vi "Extract Msg Segments.vi"(7 "Start Index":i32, 8 "error in (no error)":errorcluster, 10 "Segments in":T1[](array[typedef]), 11 "ProtoParser in":refnum<class "ProtoParser.lvclass">) -> (0 "error out":errorcluster, 1 "Message Segments":T1[](array[typedef]), 2 "Remaining":T1[](array[typedef]), 3 "ProtoParser out":refnum<class "ProtoParser.lvclass">, 5 "Next Index":i32)   [LabVIEW 2024, in "LV-Protoc.lvlib" / "ProtoParser.lvclass"]
uses:
  ProtoParser.lvclass
  ProtoParser.lvclass/ProtoParser.ctl
  Segment Type.ctl
  LV-Protoc.lvlib
  Raw Segment.ctl
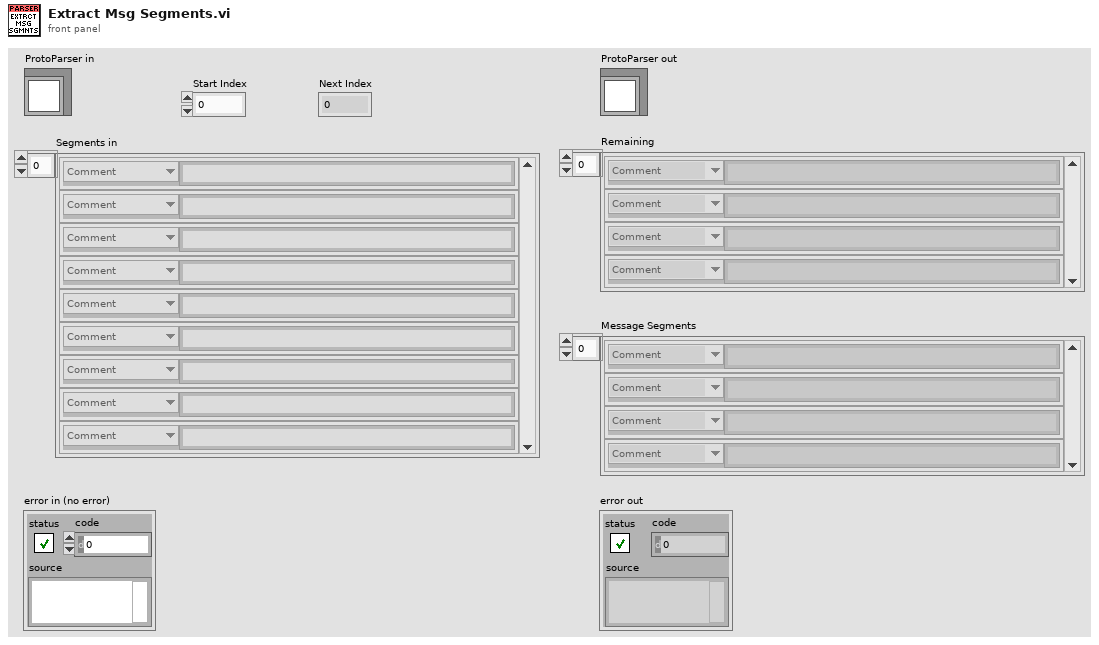
[diagram p1: front panel]
types:
  T1 = typedef "LV-Protoc.lvlib/Raw Segment.ctl" = cluster{"Type":T2, "Text":string}
  T2 = typedef "LV-Protoc.lvlib/Segment Type.ctl" = enum16{"Comment", "Message Open", "Enum Open", "Message Close", "Enum Close", "Field", "Syntax", "Import", "Enum Value", "Package", "Reserved"}
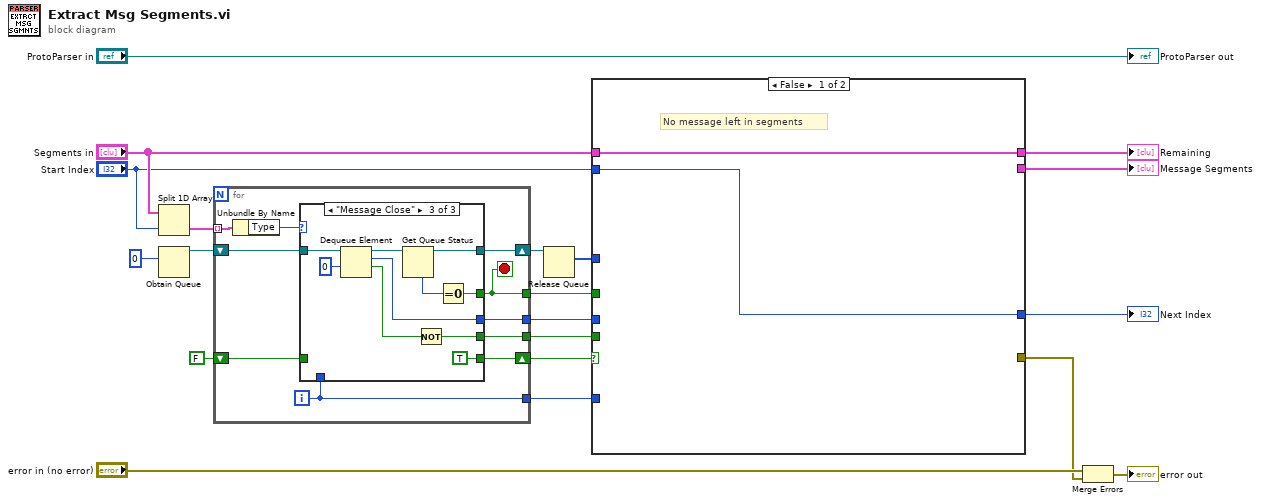
[diagram p0: block diagram]
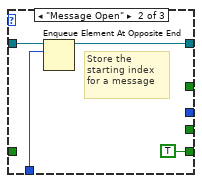
[diagram p3: hidden frame]
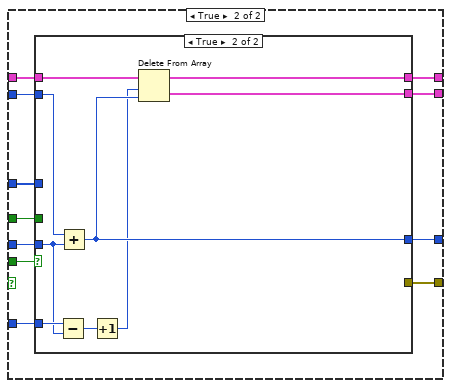
[diagram p4: hidden frame]
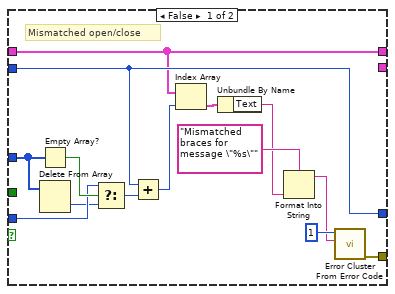
[diagram p5: hidden frame]
diagram:
  n1 = Split 1D Array(array="Segments in", index="Start Index") -> (second subarray=w16:T1[])  [unwired: 1 out]
  n2 = Obtain Queue(element data type=0) -> (queue out=w15:refnum<queue>)  [unwired: 4 in, 2 out]
  n3 = for {
    tunnel: w16 -> [w30] mode=indexing
    shift-right: [w27] -> w5
    shift-left: w15 -> [w28]
    tunnel: [w26] -> w13
    tunnel: [w25] -> w14
    tunnel: [w24] -> w11
    tunnel: [w23] -> w6
    shift-right: [w22] -> w1
    shift-left: FALSE -> [w21]
    i -> [w24]
    stop <- w23 stop-if-true
    n4 = Unbundle By Name(w30) -> ("Type"=w29:T2)
    n5 = case shown="\"Message Close\"" w29 {
      tunnel: w28 -> [w32 w35 w46]
      tunnel: [w32 w36 w44] -> w27
      tunnel: w24 -> [_ w34 _]
      tunnel: [_ _ w41] -> w23
      tunnel: [_ _ w40] -> w26
      tunnel: [_ _ w38] -> w25
      tunnel: [w31 TRUE TRUE] -> w22
      tunnel: w21 -> [w31 _ _]
      frame Default {
      }
      frame "Message Open" {
        # "Store the starting index for a message"
        n6 = Enqueue Element At Opposite End(queue=w35, element=w34) -> (queue out=w36:refnum<queue>)  [unwired: 2 in, 2 out]
      }
      frame "Message Close" {
        n7 = Dequeue Element(queue=w46, timeout in ms (-1)=0) -> (queue out=w45:refnum<queue>, element=w40:i32, timed out?=w39:bool)  [unwired: 1 in, 1 out]
        n8 = Get Queue Status(queue=w45) -> (queue out=w44:refnum<queue>, # elements in queue=w42:i32)  [unwired: 2 in, 6 out]
        n9 = Not(x=w39) -> (.not. x?=w38:bool)
        n10 = Equal To 0?(x=w42) -> (x = 0?=w41:bool)
      }
    }
  }
  n11 = Release Queue(queue=w5) -> (remaining elements=w4:i32[])  [unwired: 2 in, 2 out]
  n12 = case shown="False" w1 {
    tunnel: w14 -> [_ w59]
    tunnel: w13 -> [_ w58]
    tunnel: "Segments in" -> [w48 w57]
    tunnel: w11 -> [_ w56]
    tunnel: "Start Index" -> [w47 w55]
    tunnel: [w48 w54] -> w9
    tunnel: [w47 w53] -> w8
    tunnel: [_ w52] -> w7
    tunnel: w6 -> [_ w51]
    tunnel: w4 -> [_ w50]
    tunnel: [_ w49] -> w3
    frame False {
      # "No message left in segments"
    }
    frame True {
      n13 = case shown="True" w59 {
        tunnel: w58 -> [w72 w80]
        tunnel: w57 -> [w65 w78]
        tunnel: w56 -> [_ w82]
        tunnel: w55 -> [w66 w79]
        tunnel: [w65 w75] -> w54
        tunnel: [w66 w77] -> w53
        tunnel: [_ w76] -> w52
        tunnel: w51 -> [_ _]
        tunnel: w50 -> [w69 _]
        tunnel: [w60 _] -> w49
        frame False {
          # "Mismatched open/close"
          n14 = Empty Array?(array=w69) -> (empty?=w73:bool)
          n15 = Delete From Array(array=w69) -> (deleted portion=w71:i32)  [unwired: 2 in, 1 out]
          n16 = Select(t=w72, s=w73, f=w71) -> (s? t:f=w70:i32)
          n17 = Add(x=w66, y=w70) -> (x+y=w67:i32)
          n18 = Index Array(array=w65, index=w67) -> (element=w68:T1)
          n19 = Unbundle By Name(w68) -> ("Text"=w63:string)
          n20 = Format Into String(format string="Mismatched braces for message \"%s\"", w63) -> (resulting string=w61:string)  [unwired: 2 in, 1 out]
          n21 = call <vilib>:"Error Cluster From Error Code.vi"("error message (\"\")"=w61, "error code (0)"=1) -> ("error out"=w60:errorcluster)  [unwired: 7 in]
        }
        frame True {
          n22 = Subtract(x=w82, y=w80) -> (x-y=w81:i32)
          n23 = Add(x=w79, y=w80) -> (x+y=w77:i32)
          n24 = Increment(x=w81) -> (x+1=w74:i32)
          n25 = Delete From Array(array=w78, length=w74, index=w77) -> (deleted portion=w76:T1[], array with subset deleted=w75:T1[])
        }
      }
    }
  }
  "Message Segments" <- w7
  "Next Index" <- w8
  "Remaining" <- w9
  n26 = Merge Errors("error in (no error)", w3) -> (→"error out":errorcluster)
  "ProtoParser out" <- "ProtoParser in"
